vi "Read.vi"(8 "Error In":errorcluster, 11 "SerialComm in":refnum<class "SerialComm.lvclass">) -> (0 "Error Out":errorcluster, 3 "SerialComm out":refnum<class "SerialComm.lvclass">)   [LabVIEW 2017, in "SerialComm.lvclass"]
uses:
  SerialComm.lvclass
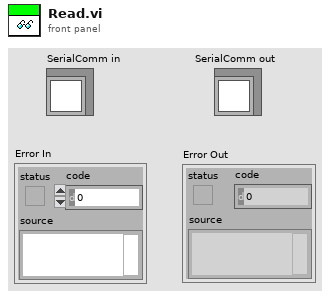
[diagram p1: front panel]
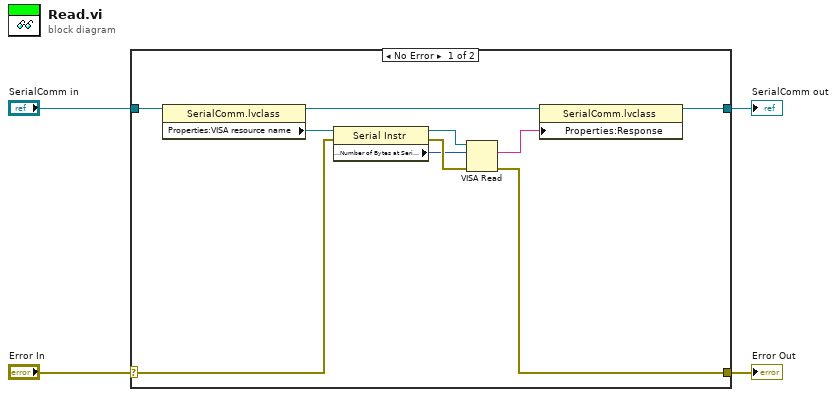
[diagram p0: block diagram]
diagram:
  n1 = case shown="No Error" "Error In" {
    selector: "Error In" -> [w12 w16]
    tunnel: [w9 w16] -> w3
    tunnel: [w8 w15] -> w1
    tunnel: "SerialComm in" -> [w14 w15]
    frame No Error {
      n2 = property class="SerialComm.lvclass"(reference=w14) -> (reference out=w13:refnum<class "SerialComm.lvclass">, "Properties:VISA resource name"=w5:refnum<visa-resource-name>)  [unwired: 1 in, 1 out]
      n3 = property class="Serial Instr"(reference=w5, error in=w12) -> (reference out=w11:refnum<visa-resource-name>, error out=w10:errorcluster, "Serial Settings:Number of Bytes at Serial Port"=w6:u32)
      n4 = VISA Read(VISA resource name=w11, byte count=w6, error in (no error)=w10) -> (read buffer=w7:string, error out=w9:errorcluster)  [unwired: 2 out]
      n5 = property class="SerialComm.lvclass"(reference=w13, "Properties:Response"=w7) -> (reference out=w8:refnum<class "SerialComm.lvclass">)  [unwired: 1 in, 1 out]
    }
    frame Error {
    }
  }
  "Error Out" <- w3
  "SerialComm out" <- w1
